vi "Pos timeout.vi"(7 "AI Parameters":T1={"GotoKick"={"Dist do cone a frente"=150.0, "attacker farback"=1500.0, "Perto"=300.0, "min dist to kick"=150.0, "kick eps"=0.0, "Time to transition"=0.05}, "Attacker"={"CC chute"=0.09, "CC passe"=0.045, "Kick Force"=100.0, "D ball-robot Kick"=200.0, "D ball-robot Pass"=0.3}, "Defender"={"D max"=1700.0, "Vel p/ robô av"=1000.0, "Kick Force"=100.0, "D atk-def"=0.0, "D farback"=0.0}, "Timeout"={"Field/v in x"=6.0, "Dist Robots"=300, "Dist up in y"=300}, "Pose Striker"={"dist"=200.0, "Numeric"=-4.0, "dist 2"=200.0}, "Dist Stop"=300.0, "Distance when ball out"=200, "D central gap "=150.0, "T pass"=0.0, "Force ++"=0.0, "range kick"=0.0, "Chute alto"=TRUE, "Marcador novo"=TRUE} {"D central gap" format="%#_13g"; "Dist Stop" format="%#_13g"; "Pose Striker"."Numeric" format="%#_13g"; "Defender"."Kick Force" format="%#_13g"; "Defender"."Vel p/ robô av" format="%#_13g"; "Attacker"."D ball-robot Kick" format="%#_13g"; "Attacker"."Kick Force" format="%#_13g"; "Attacker"."CC passe" format="%#_13g"; "Attacker"."CC chute" format="%#_13g"; "GotoKick"."kick eps" format="%#_13g"; "GotoKick"."min dist to kick" format="%#_13g"; "GotoKick"."Perto" format="%#_13g"; "GotoKick"."attacker farback" format="%#_13g"; "GotoKick"."Dist do cone a frente" format="%#_13g"}, 9 "robos":u32[](array[numeric]), 10 "IA State Input":T2={"our_robots"=[], "enemy_robots"=[], "balls"=[], "geometry"={"line_width"=0, "field_length"=0, "field_width"=0, "boundary_width"=0, "referee_width"=0, "goal_width"=0, "goal_depth"=0, "goal_wall_width"=0, "center_circle_radius"=0, "defense_radius"=0, "defense_stretch"=0, "free_kick_from_defense_dist"=0, "penalty_spot_from_field_line_dist"=0, "penalty_line_from_spot_dist"=0}, "IA Judge"={"stage"="", "command"="", "our_goalie_id"=0.0, "enemy_goalie_id"=0.0, "command enum"=enum."Halt", "Time"=enum."Azul"}, "Received Timestamp"=timestamp(0 s since 1904-01-01), "Events"={"Touch"=FALSE, "Ball out"=FALSE, "id touch"=0.0, "Ball out of \nVision"=FALSE, "Ball inside \nGoalie area"=FALSE, "Robot not responding"=FALSE, "Robots responding status"=[1.0, 1.0, 1.0, 1.0, 1.0, 1.0], "Enemy Ball \nPossession"=FALSE, "Pass State"=FALSE, "id end of pass"=0.0, "Kick"=FALSE, "Id ini Possession"=0.0, "Ball Possesion"=FALSE, "Id Possesion"=0.0}}) -> (2 "Posição dos robos":dbl[][](array[numeric]))   [LabVIEW 2017]
uses:
  Core/AI Input.ctl
  Core/AI Robot.ctl
  Functions Enum.ctl
  AttackerStates.ctl
  Core/AI Ball.ctl
  Core/Field Size.ctl
  Core/AI Judge.ctl
  Command Enum.ctl
  Util/Events/Events.ctl
  AI Parameters.ctl
panel:
  in  "Array  in":dbl[][](array[numeric])=[[99999.0, 99999.0], [99999.0, 99999.0], [99999.0, 99999.0], [99999.0, 99999.0], [99999.0, 99999.0], [99999.0, 99999.0], [99999.0, 99999.0]]
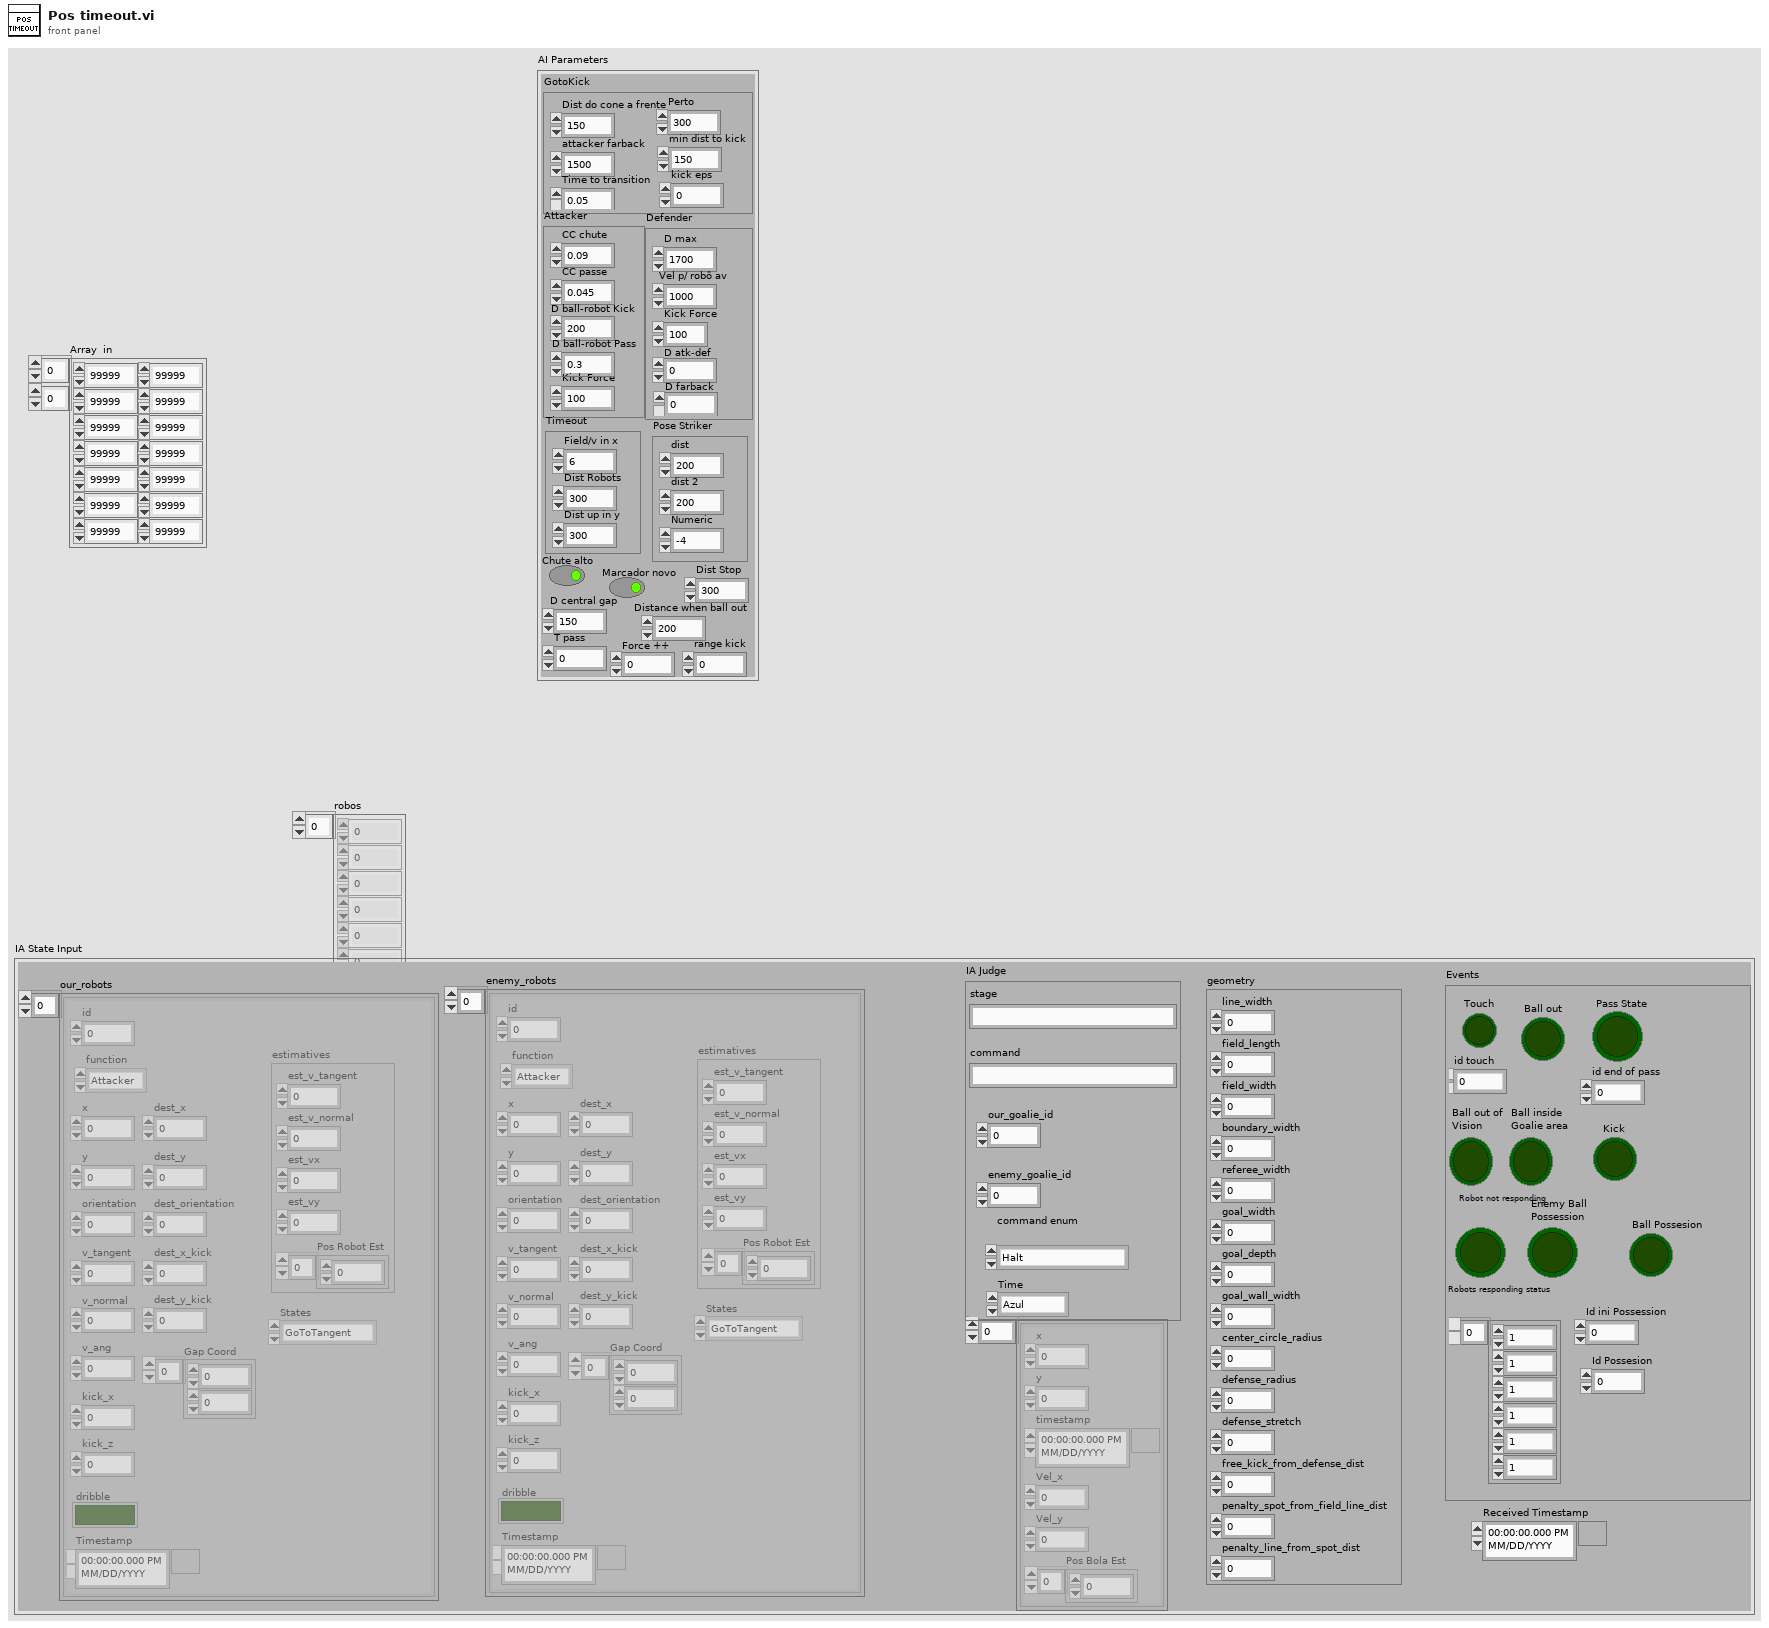
[diagram p1: front panel]
types:
  T1 = typedef "AI Parameters.ctl" = cluster{"GotoKick":cluster{"Dist do cone a frente":dbl, "attacker farback":dbl, "Perto":dbl, "min dist to kick":dbl, "kick eps":dbl, "Time to transition":dbl}, "Attacker":cluster{"CC chute":dbl, "CC passe":dbl, "Kick Force":dbl, "D ball-robot Kick":dbl, "D ball-robot Pass":dbl}, "Defender":cluster{"D max":dbl, "Vel p/ robô av":dbl, "Kick Force":dbl, "D atk-def":dbl, "D farback":dbl}, "Timeout":cluster{"Field/v in x":dbl, "Dist Robots":u32, "Dist up in y":u32}, "Pose Striker":cluster{"dist":dbl, "Numeric":dbl, "dist 2":dbl}, "Dist Stop":dbl, "Distance when ball out":i32, "D central gap ":dbl, "T pass":dbl, "Force ++":dbl, "range kick":dbl, "Chute alto":bool, "Marcador novo":bool}
  T2 = typedef "AI Input.ctl" = cluster{"our_robots":T3[], "enemy_robots":T3[], "balls":T6[], "geometry":T7, "IA Judge":T8, "Received Timestamp":timestamp, "Events":T10}
  T3 = typedef "AI Robot.ctl" = cluster{"id":u32, "function":T4, "x":dbl, "y":dbl, "orientation":dbl, "v_tangent":dbl, "v_normal":dbl, "v_ang":dbl, "kick_x":dbl, "kick_z":dbl, "dribble":bool, "Timestamp":timestamp, "dest_x":dbl, "dest_y":dbl, "dest_orientation":dbl, "estimatives":cluster{"est_v_tangent":dbl, "est_v_normal":dbl, "est_vx":dbl, "est_vy":dbl, "Pos Robot Est":dbl[]}, "dest_x_kick":dbl, "dest_y_kick":dbl, "Gap Coord":dbl[], "States":T5}
  T4 = typedef "Functions Enum.ctl" = enum16{"Attacker", "Goalie", "Defender", "Striker", "Goto 0", "Dummy", "Kicker", "ZigZag"}
  T5 = typedef "AttackerStates.ctl" = enum16{"Pass", "GoToTangent", "BallGetting", "GoToKick", ""}
  T6 = typedef "AI Ball.ctl" = cluster{"x":dbl, "y":dbl, "timestamp":timestamp, "Vel_x":dbl, "Vel_y":dbl, "Pos Bola Est":dbl[]}
  T7 = typedef "Field Size.ctl" = cluster{"line_width":u32, "field_length":u32, "field_width":u32, "boundary_width":u32, "referee_width":u32, "goal_width":u32, "goal_depth":u32, "goal_wall_width":u32, "center_circle_radius":u32, "defense_radius":u32, "defense_stretch":u32, "free_kick_from_defense_dist":u32, "penalty_spot_from_field_line_dist":u32, "penalty_line_from_spot_dist":u32}
  T8 = typedef "AI Judge.ctl" = cluster{"stage":string, "command":string, "our_goalie_id":dbl, "enemy_goalie_id":dbl, "command enum":T9, "Time":enum16{"Azul", "Amarelo"}}
  T9 = typedef "Command Enum.ctl" = enum16{"Halt", "Stop", "Force Start", "PKA Normal Start", "Prepare Kickoff Ally", "PKE Normal Start", "Prepare Kickoff Enemy", "Prepare Penalty Ally", "PPA Normal Start", "Prepare Penalty Enemy", "PPE Normal Start", "Direct Free Enemy", "Direct Free Ally", "Indirect Free Enemy", "Indirect Free Ally", "Timeout Enemy", "Timeout Ally", "Goal Enemy", "Goal Ally", "Ball Placement Enemy", "Ball Placement Ally", "Normal Half Time", "Extra Time Break", "Extra Half Time", "None", "Post Game"}
  T10 = typedef "Events.ctl" = cluster{"Touch":bool, "Ball out":bool, "id touch":dbl, "Ball out of \nVision":bool, "Ball inside \nGoalie area":bool, "Robot not responding":bool, "Robots responding status":dbl[], "Enemy Ball \nPossession":bool, "Pass State":bool, "id end of pass":dbl, "Kick":bool, "Id ini Possession":dbl, "Ball Possesion":bool, "Id Possesion":dbl}
  T11 = cluster{"Field/v in x":dbl, "Dist Robots":u32, "Dist up in y":u32}
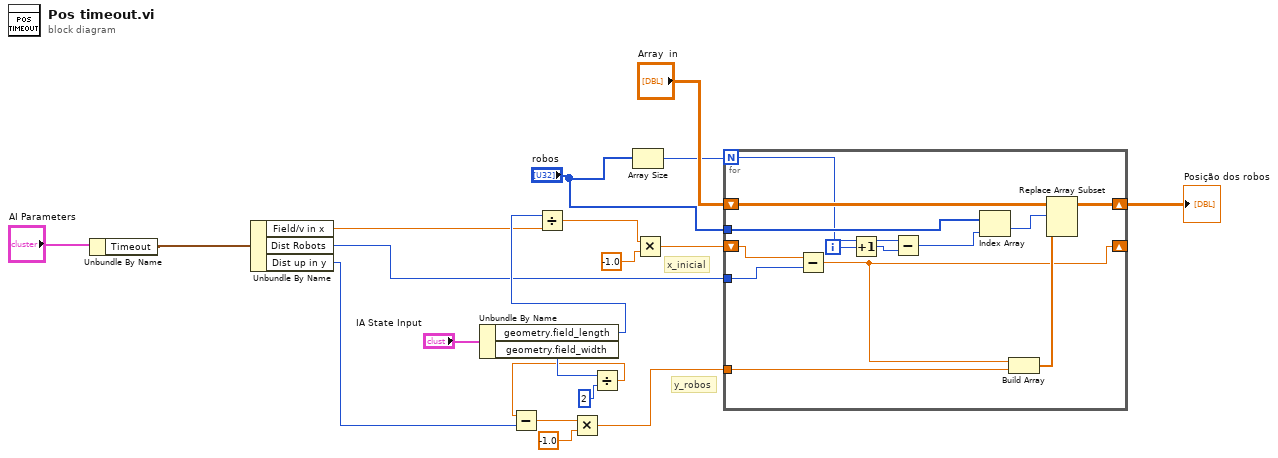
[diagram p0: block diagram]
diagram:
  # "x_inicial"
  # "y_robos"
  n1 = Unbundle By Name("AI Parameters") -> ("Timeout"=w1:T11)
  n2 = Unbundle By Name(w1) -> ("Field/v in x"=w5:dbl, "Dist Robots"=w4:u32, "Dist up in y"=w3:u32)
  n3 = Unbundle By Name("IA State Input") -> ("geometry.field_length"=w14:u32, "geometry.field_width"=w11:u32)
  n4 = Divide(x=w14, y=w5) -> (x/y=w13:dbl)
  n5 = Divide(x=w11, y=u32 2) -> (x/y=w10:dbl)
  n6 = Subtract(x=w10, y=w3) -> (x-y=w18:dbl)
  n7 = Multiply(x=w18, y=-1.0) -> (x*y=w8:dbl)
  n8 = Array Size(array="robos") -> (size(s)=w7:i32)
  n9 = Multiply(x=w13, y=-1.0) -> (x*y=w9:dbl)
  n10 = for {
    N: w7 -> [w24]
    shift-right: [w31] -> w20
    shift-left: "Array  in" -> [w32]
    shift-right: [w27] -> _
    shift-left: w9 -> [w28]
    tunnel: w8 -> [w29]
    tunnel: "robos" -> [w26]
    tunnel: w4 -> [w25]
    i -> [w22]
    n11 = Subtract(x=w28, y=w25) -> (x-y=w27:dbl)
    n12 = Increment(x=w22) -> (x+1=w21:i32)
    n13 = Subtract(x=w24, y=w21) -> (x-y=w23:i32)
    n14 = Index Array(array=w26, index=w23) -> (element=w33:u32)
    n15 = Build Array(w27, w29) -> (w30:dbl[])
    n16 = Replace Array Subset(array=w32, new element=w30, index (row)=w33) -> (w31:dbl[][])  [unwired: 1 in]
  }
  "Posição dos robos" <- w20
